vi "StartAsync.vi"(4 "ErrorQueue":refnum<queue>, 7 "Actor in":refnum<class "Actor.lvclass">, 8 "Error in":errorcluster) -> (0 "Error out":errorcluster)   [LabVIEW 2020, in "jettl.lvlib"]
uses:
  jettl.lvlib
  Actor.vi
  Actor/Actor.lvclass
  Message/Message.lvclass
  Msg Contents/Msg Contents.lvclass
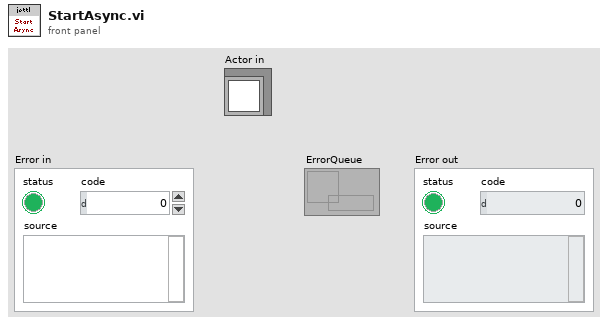
[diagram p1: front panel]
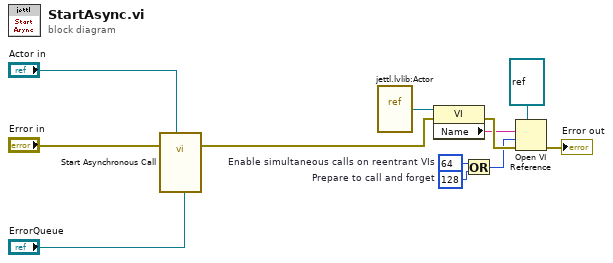
[diagram p0: block diagram]
diagram:
  w4 = 64  # Enable simultaneous calls on reentrant VIs
  w5 = 128  # Prepare to call and forget
  n1 = call-by-ref "Start Asynchronous Call"(error in="Error in", "ErrorQueue"="ErrorQueue", "Actor in"="Actor in") -> (error out=w1:errorcluster)  [unwired: 9 in, 3 out]
  n2 = vi-ref "jettl.lvlib:Actor.vi"() -> (w7:refnum<vi>)
  n3 = property class="VI"(reference=w7, error in=w1) -> (error out=w9:errorcluster, "Name"=w8:string)  [unwired: 1 out]
  n4 = Or(x=w4, y=w5) -> (x .or. y?=w3:i32)
  n5 = Open VI Reference(type specifier VI Refnum (for type only)=refnum<vi> refnum, vi path=w8, options=w3, error in (no error)=w9) -> (error out=→"Error out":errorcluster)  [unwired: 2 in, 1 out]
